vi "Queue.vi"() -> ()   [LabVIEW 2014]
panel:
  in  "milliseconds to wait":u32=4
  out "Enqueued Element":dynamicdata(graph)
  in  "Stop 2":bool
  out "Elements in Queue":i32(slide) scale=0.0..10.0
  out "Numeric":dbl
  out "Phase 2":dbl
  out "Frequency 2":dbl
  out "Amplitude 2":dbl
  out "Phase":dbl
  out "Frequency":dbl
  out "Amplitude":dbl
  out "Dequeued elements":dynamicdata(graph)
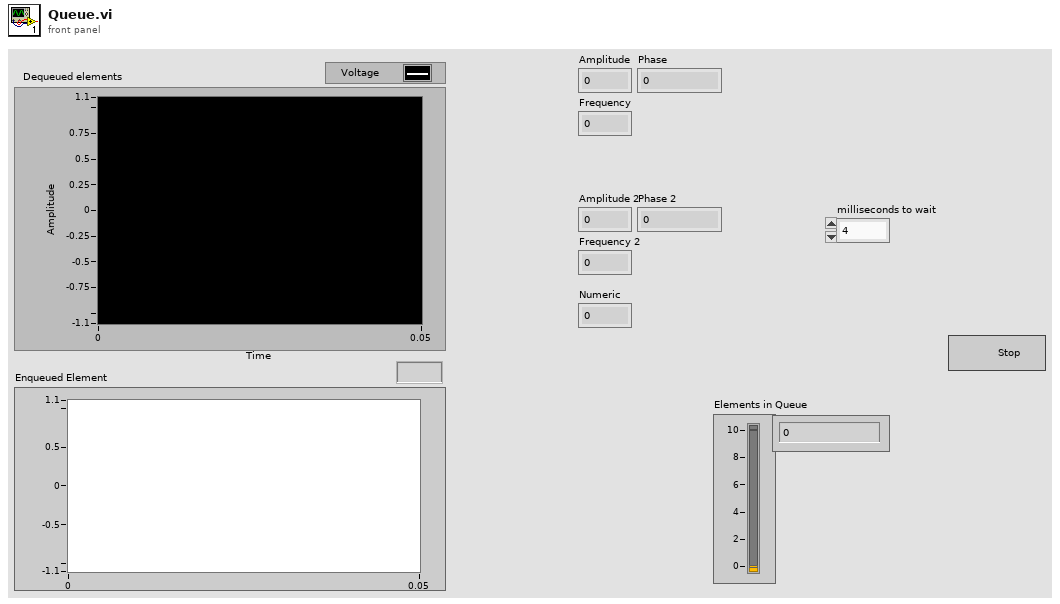
[diagram p1: front panel]
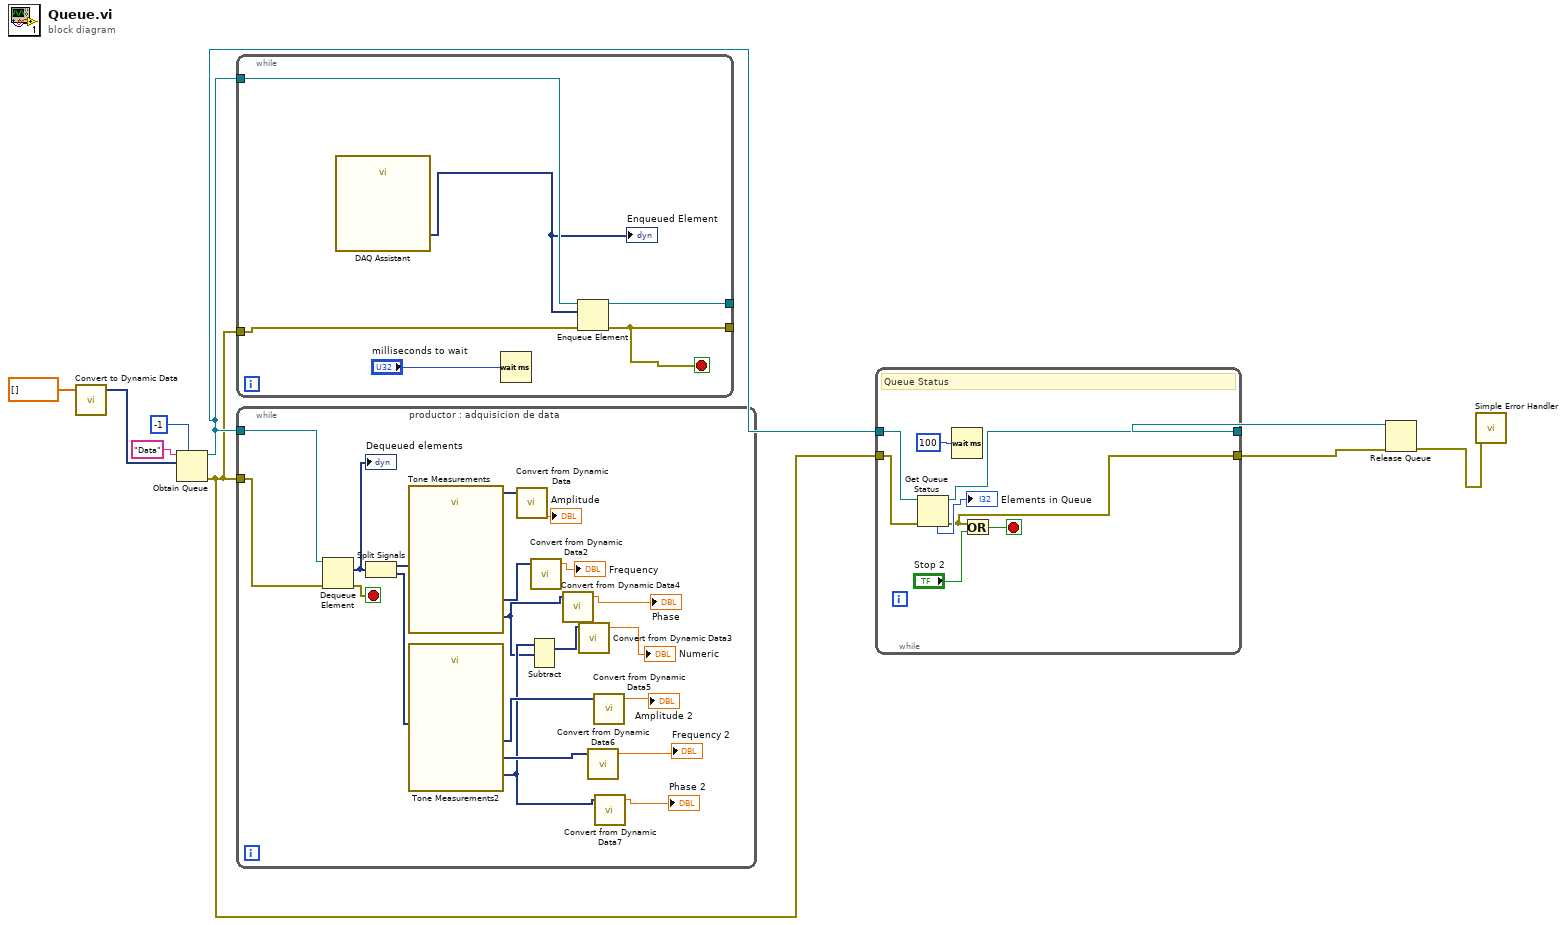
[diagram p0: block diagram]
diagram:
  n1 = call "Convert to Dynamic Data"("Array"=dbl[] []) -> ("Dynamic Data Type"=w9:dynamicdata)  [unwired: 3 in]
  n2 = Obtain Queue(max queue size (-1, unlimited)=-1, name (unnamed)="Data", element data type=w9) -> (queue out=w5:refnum<queue>, error out=w3:errorcluster)  [unwired: 2 in, 1 out]
  n3 = while "productor : adquisicion de data" {
    tunnel: w5 -> [w15]
    tunnel: [w14] -> _
    tunnel: w3 -> [w13]
    tunnel: [w12] -> _
    stop <- w12 stop-if-true
    n4 = call "DAQ Assistant"() -> ("data"=w10:dynamicdata)  [unwired: 16 in, 3 out]
    "Enqueued Element" <- w10
    n5 = Wait (ms)(milliseconds to wait="milliseconds to wait") -> ()  [unwired: 1 out]
    n6 = Enqueue Element(queue=w15, element=w10, error in (no error)=w13) -> (queue out=w14:refnum<queue>, error out=w12:errorcluster)  [unwired: 1 in, 1 out]
  }
  n7 = while {
    tunnel: w5 -> [w35]
    tunnel: w3 -> [w31]
    stop <- w30 stop-if-true
    n8 = Dequeue Element(queue=w35, error in (no error)=w31) -> (element=w34:dynamicdata, error out=w30:errorcluster)  [unwired: 1 in, 2 out]
    "Dequeued elements" <- w34
    n9 = Split Signals(w34) -> (w33:dynamicdata, w32:dynamicdata)  [unwired: 2 in]
    n10 = call "Tone Measurements"("Signals"=w33) -> ("Phase"=w19:dynamicdata, "Frequency"=w27:dynamicdata, "Amplitude"=w29:dynamicdata)  [unwired: 7 in, 1 out]
    n11 = call "Tone Measurements2"("Signals"=w32) -> ("Phase"=w21:dynamicdata, "Frequency"=w23:dynamicdata, "Amplitude"=w25:dynamicdata)  [unwired: 7 in, 1 out]
    n12 = call "Convert from Dynamic Data"("Dynamic Data Type"=w29) -> ("Scalar"=→"Amplitude":dbl)  [unwired: 3 in]
    n13 = Subtract(1:w19, 2:w21) -> (0:w17:dynamicdata)  [unwired: 1 in, 1 out]
    n14 = call "Convert from Dynamic Data2"("Dynamic Data Type"=w27) -> ("Scalar"=→"Frequency":dbl)  [unwired: 3 in]
    n15 = call "Convert from Dynamic Data4"("Dynamic Data Type"=w19) -> ("Scalar"=→"Phase":dbl)  [unwired: 3 in]
    n16 = call "Convert from Dynamic Data3"("Dynamic Data Type"=w17) -> ("Scalar"=→"Numeric":dbl)  [unwired: 3 in]
    n17 = call "Convert from Dynamic Data6"("Dynamic Data Type"=w23) -> ("Scalar"=→"Frequency 2":dbl)  [unwired: 3 in]
    n18 = call "Convert from Dynamic Data5"("Dynamic Data Type"=w25) -> ("Scalar"=→"Amplitude 2":dbl)  [unwired: 3 in]
    n19 = call "Convert from Dynamic Data7"("Dynamic Data Type"=w21) -> ("Scalar"=→"Phase 2":dbl)  [unwired: 3 in]
  }
  n20 = while {
    tunnel: w5 -> [w43]
    tunnel: [w37] -> w2
    tunnel: w3 -> [w39]
    tunnel: [w38] -> w1
    stop <- w41 stop-if-true
    # "Queue Status"
    n21 = Get Queue Status(queue=w43, error in (no error)=w39) -> (queue out=w38:refnum<queue>, error out=w37:errorcluster, # elements in queue=→"Elements in Queue":i32)  [unwired: 6 out]
    n22 = Wait (ms)(milliseconds to wait=u32 100) -> ()  [unwired: 1 out]
    n23 = Or(x=w37, y="Stop 2") -> (x .or. y?=w41:bool)
  }
  n24 = Release Queue(queue=w1, error in (no error)=w2) -> (error out=w4:errorcluster)  [unwired: 1 in, 2 out]
  n25 = call <vilib>:"Simple Error Handler.vi"("error in (no error)"=w4) -> ()  [unwired: 1 in, 8 out]
